vi "Motor_Cascade_Strage.vi"(0 "P1_Value":T1=enum."Off", 1 "P1_Enable":bool, 2 "P3_Enable":bool, 5 "P2_Value":T1=enum."Off", 7 "P3_Value":T1=enum."Off", 9 "P4_Value":T1=enum."Off", 12 "P2_Enable":bool, 13 "P4_Enable":bool) -> (4 "P Out":T1, 6 "Any True?":bool)   [LabVIEW 2015]
uses:
  Motor_Dir_Type_Def.ctl
panel:
  # "P1 is highest priority\np5 is lowest"
  # "Josh Merkle 2/8/16"
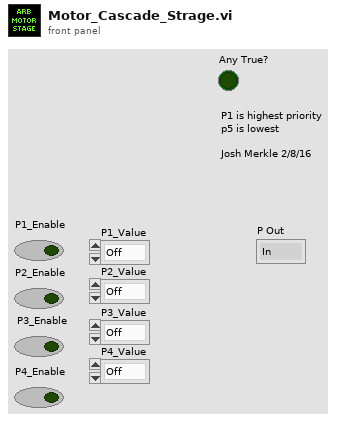
[diagram p1: front panel]
types:
  T1 = typedef "Motor_Dir_Type_Def.ctl" = enum16{"In", "Out", "Off"}
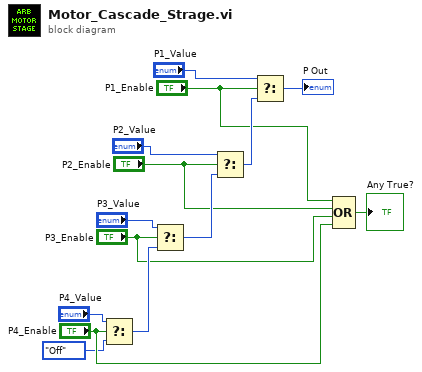
[diagram p0: block diagram]
diagram:
  n1 = Select(t="P4_Value", s="P4_Enable", f=Motor_Dir_Type_Def."Off" ("P2_Value 2")) -> (s? t:f=w14:T1)
  n2 = Select(t="P3_Value", s="P3_Enable", f=w14) -> (s? t:f=w13:T1)
  n3 = Select(t="P2_Value", s="P2_Enable", f=w13) -> (s? t:f=w12:T1)
  n4 = Select(t="P1_Value", s="P1_Enable", f=w12) -> (s? t:f=→"P Out":T1)
  n5 = Compound Arithmetic op=OR("P1_Enable", "P2_Enable", "P3_Enable", "P4_Enable") -> (→"Any True?":bool)
